vi "MovingAverage.vi"(0 "Moving average":dbl, 7 "Random number":dbl, 11 "Error in":errorcluster) -> (4 "Average":dbl, 15 "Error out":errorcluster)   [LabVIEW 2020]
uses:
  <vilib>/Analysis/baseanly.llb/Mean (DBL).vi
  <vilib>/Analysis/NI_AALBase.lvlib
panel:
  out "Generated array":dbl[](array[numeric])
  # "INPUT"
  # "OUTPUT"
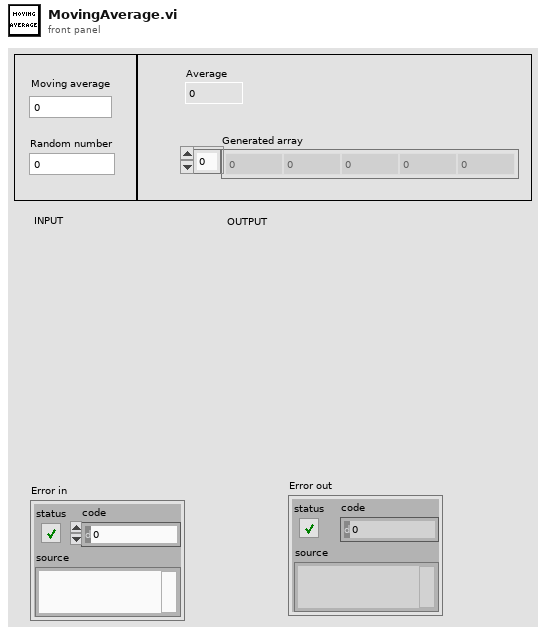
[diagram p1: front panel]
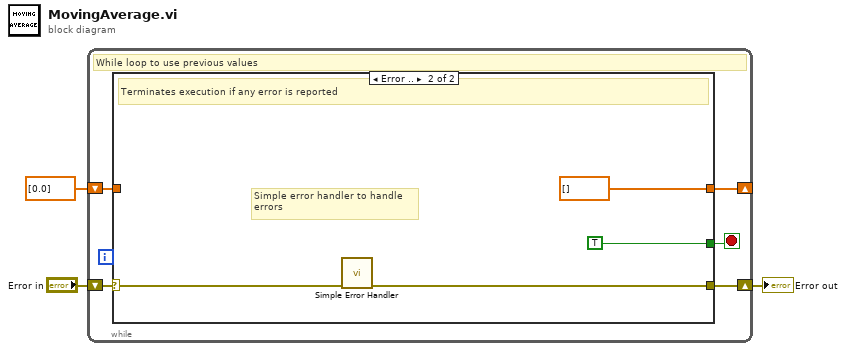
[diagram p0: block diagram]
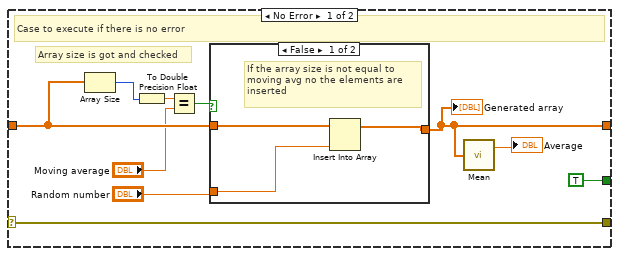
[diagram p2: hidden frame]
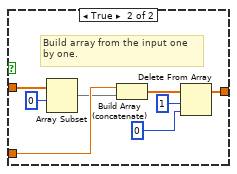
[diagram p3: hidden frame]
diagram:
  n1 = while {
    shift-right: [w7] -> w2
    shift-left: "Error in" -> [w8]
    shift-right: [w5] -> _
    shift-left: dbl[] [0.0] -> [w4]
    stop <- w6 stop-if-true
    # "While loop to use previous values"
    n2 = case shown="Error .." w8 {
      selector: w8 -> [w18 w31]
      tunnel: [w18 w30] -> w7
      tunnel: [TRUE TRUE] -> w6
      tunnel: [w9 dbl[] []] -> w5
      tunnel: w4 -> [w15 _]
      frame No Error {
        # "Array size is got and checked"
        # "Case to execute if there is no error"
        n3 = Array Size(array=w15) -> (size(s)=w11:i32)
        n4 = To Double Precision Float(number=w11) -> (double precision float=w12:dbl)
        n5 = Equal?(x=w12, y="Moving average") -> (x = y?=w17:bool)
        n6 = case shown="False" w17 {
          tunnel: [w21 w24] -> w9
          tunnel: w15 -> [w20 w29]
          tunnel: "Random number" -> [w19 w27]
          frame False {
            # "If the array size is not equal to \nmoving avg no the elements are \ninserted"
            n7 = Insert Into Array(array=w20, new element=w19) -> (w21:dbl[])  [unwired: 1 in]
          }
          frame True {
            # "Build array from the input one\nby one."
            n8 = Array Subset(array=w29, index=0) -> (w26:dbl[])  [unwired: 1 in]
            n9 = Build Array (concatenate)(w27, w26) -> (w25:dbl[])
            n10 = Delete From Array(array=w25, length=1, index=0) -> (array with subset deleted=w24:dbl[])  [unwired: 1 out]
          }
        }
        "Generated array" <- w9
        n11 = call-poly <vilib>:"Mean.vi"("X"=w9) -> ("mean"=→"Average":dbl)  [unwired: 1 out]
      }
      frame Error {
        # "Simple error handler to handle \nerrors"
        # "Terminates execution if any error is reported"
        n12 = call <vilib>:"Simple Error Handler.vi"("error in (no error)"=w31) -> ("error out"=w30:errorcluster)  [unwired: 4 in, 4 out]
      }
    }
  }
  "Error out" <- w2
